vi "GeoData.vi"() -> ()   [LabVIEW 2017] (continued)
County\tH4\n1063\t25015\tNorthampton\tMA\tHampshire County\tH4\n1066\t25015\tNorth hatfield\tMA\tHampshire County\tH4\n1243\t25015\tMiddlefield\tMA\tHampshire County\tH4\n1007\t25015\tBelchertown\tMA\tHampshire County\tH4\n1011\t25015\tChester\tMA\tHampshire County\tH4\n1012\t25015\tChesterfield\tMA\tHampshire County\tH4\n1032\t25015\tGoshen\tMA\tHampshire County\tH4\n1027\t25015\tEasthampton\tMA\tHampshire County\tH4\n1060\t25015\tNorthampton\tMA\tHampshire County\tH4\n1033\t25015\tGranby\tMA\tHampshire County\tH4\n1038\t25015\tHatfield\tMA\tHampshire County\tH4\n1462\t25017\tLunenburg\tMA\tMiddlesex County\tH4\n1464\t25017\tShirley\tMA\tMiddlesex County\tH4\n1776\t25017\tSudbury\tMA\tMiddlesex County\tH4\n1803\t25017\tBurlington\tMA\tMiddlesex County\tH4\n1810\t25017\tAndover\tMA\tMiddlesex County\tH4\n1854\t25017\tLowell\tMA\tMiddlesex County\tH4\n1862\t25017\tNorth billerica\tMA\tMiddlesex County\tH4\n1879\t25017\tTyngsboro\tMA\tMiddlesex County\tH4\n2030\t25017\tDover\tMA\tMiddlesex County\tH4\n2054\t25017\tMillis\tMA\tMiddlesex County\tH4\n2143\t25017\tSomerville\tMA\tMiddlesex County\tH4\n2476\t25017\tArlington\tMA\tMiddlesex County\tH4\n1853\t25017\tLowell\tMA\tMiddlesex County\tH4\n1469\t25017\tTownsend\tMA\tMiddlesex County\tH4\n1703\t25017\tFramingham\tMA\tMiddlesex County\tH4\n1784\t25017\tWoodville\tMA\tMiddlesex County\tH4\n1805\t25017\tBurlington\tMA\tMiddlesex County\tH4\n1460\t25017\tLittleton\tMA\tMiddlesex County\tH4\n1746\t25017\tHolliston\tMA\tMiddlesex County\tH4\n1850\t25017\tLowell\tMA\tMiddlesex County\tH4\n1865\t25017\tNutting lake\tMA\tMiddlesex County\tH4\n1867\t25017\tReading\tMA\tMiddlesex County\tH4\n1876\t25017\tTewksbury\tMA\tMiddlesex County\tH4\n1880\t25017\tWakefield\tMA\tMiddlesex County\tH4\n1887\t25017\tWilmington\tMA\tMiddlesex County\tH4\n2149\t25017\tEverett\tMA\tMiddlesex County\tH4\n2238\t25017\tCambridge\tMA\tMiddlesex County\tH4\n2453\t25017\tWaltham\tMA\tMiddlesex County\tH4\n2454\t25017\tWaltham\tMA\tMiddlesex County\tH4\n2466\t25017\tAuburndale\tMA\tMiddlesex County\tH4\n1752\t25017\tMarlborough\tMA\tMiddlesex County\tH4\n1749\t25017\tHudson\tMA\tMiddlesex County\tH4\n1778\t25017\tWayland\tMA\tMiddlesex County\tH4\n2138\t25017\tCambridge\tMA\tMiddlesex County\tH4\n2142\t25017\tCambridge\tMA\tMiddlesex County\tH4\n2145\t25017\tSomerville\tMA\tMiddlesex County\tH4\n2151\t25017\tRevere\tMA\tMiddlesex County\tH4\n2452\t25017\tWaltham\tMA\tMiddlesex County\tH4\n2465\t25017\tWest newton\tMA\tMiddlesex County\tH4\n2461\t25017\tNewton highlands\tMA\tMiddlesex County\tH4\n2474\t25017\tArlington\tMA\tMiddlesex County\tH4\n2471\t25017\tWatertown\tMA\tMiddlesex County\tH4\n1718\t25017\tActon\tMA\tMiddlesex County\tH4\n1866\t25017\tPinehurst\tMA\tMiddlesex County\tH4\n1432\t25017\tAyer\tMA\tMiddlesex County\tH4\n1431\t25017\tAshby\tMA\tMiddlesex County\tH4\n1451\t25017\tHarvard\tMA\tMiddlesex County\tH4\n1701\t25017\tFramingham\tMA\tMiddlesex County\tH4\n1730\t25017\tBedford\tMA\tMiddlesex County\tH4\n1801\t25017\tWoburn\tMA\tMiddlesex County\tH4\n1822\t25017\tBillerica\tMA\tMiddlesex County\tH4\n2140\t25017\tCambridge\tMA\tMiddlesex County\tH4\n2459\t25017\tNewton center\tMA\tMiddlesex County\tH4\n1463\t25017\tPepperell\tMA\tMiddlesex County\tH4\n1474\t25017\tWest townsend\tMA\tMiddlesex County\tH4\n1720\t25017\tActon\tMA\tMiddlesex County\tH4\n1742\t25017\tConcord\tMA\tMiddlesex County\tH4\n1821\t25017\tBillerica\tMA\tMiddlesex County\tH4\n1851\t25017\tLowell\tMA\tMiddlesex County\tH4\n1863\t25017\tNorth chelmsford\tMA\tMiddlesex County\tH4\n2148\t25017\tMalden\tMA\tMiddlesex County\tH4\n2150\t25017\tChelsea\tMA\tMiddlesex County\tH4\n1741\t25017\tCarlisle\tMA\tMiddlesex County\tH4\n2462\t25017\tNewton lower falls\tMA\tMiddlesex County\tH4\n1472\t25017\tWest groton\tMA\tMiddlesex County\tH4\n2477\t25017\tWatertown\tMA\tMiddlesex County\tH4\n1532\t25017\tNorthborough\tMA\tMiddlesex County\tH4\n1721\t25017\tAshland\tMA\tMiddlesex County\tH4\n1748\t25017\tHopkinton\tMA\tMiddlesex County\tH4\n1760\t25017\tNatick\tMA\tMiddlesex County\tH4\n1770\t25017\tSherborn\tMA\tMiddlesex County\tH4\n1826\t25017\tDracut\tMA\tMiddlesex County\tH4\n1886\t25017\tWestford\tMA\tMiddlesex County\tH4\n2176\t25017\tMelrose\tMA\tMiddlesex County\tH4\n2451\t25017\tWaltham\tMA\tMiddlesex County\tH4\n2467\t25017\tChestnut hill\tMA\tMiddlesex County\tH4\n2478\t25017\tBelmont\tMA\tMiddlesex County\tH4\n1775\t25017\tStow\tMA\tMiddlesex County\tH4\n2464\t25017\tNewton upper falls\tMA\tMiddlesex County\tH4\n1824\t25017\tChelmsford\tMA\tMiddlesex County\tH4\n1827\t25017\tDunstable\tMA\tMiddlesex County\tH4\n1852\t25017\tLowell\tMA\tMiddlesex County\tH4\n1864\t25017\tNorth reading\tMA\tMiddlesex County\tH4\n2155\t25017\tMedford\tMA\tMiddlesex County\tH4\n2180\t25017\tStoneham\tMA\tMiddlesex County\tH4\n2420\t25017\tLexington\tMA\tMiddlesex County\tH4\n2460\t25017\tNewtonville\tMA\tMiddlesex County\tH4\n2472\t25017\tWatertown\tMA\tMiddlesex County\tH4\n2493\t25017\tWeston\tMA\tMiddlesex County\tH4\n1434\t25017\tDevens\tMA\tMiddlesex County\tH4\n1773\t25017\tLincoln\tMA\tMiddlesex County\tH4\n1888\t25017\tWoburn\tMA\tMiddlesex County\tH4\n2455\t25017\tNorth waltham\tMA\tMiddlesex County\tH4\n1450\t25017\tGroton\tMA\tMiddlesex County\tH4\n1702\t25017\tFramingham\tMA\tMiddlesex County\tH4\n1754\t25017\tMaynard\tMA\tMiddlesex County\tH4\n1890\t25017\tWinchester\tMA\tMiddlesex County\tH4\n1906\t25017\tSaugus\tMA\tMiddlesex County\tH4\n2139\t25017\tCambridge\tMA\tMiddlesex County\tH4\n2141\t25017\tCambridge\tMA\tMiddlesex County\tH4\n2144\t25017\tSomerville\tMA\tMiddlesex County\tH4\n2421\t25017\tLexington\tMA\tMiddlesex County\tH4\n2458\t25017\tNewton\tMA\tMiddlesex County\tH4\n1719\t25017\tBoxborough\tMA\tMiddlesex County\tH4\n2468\t25017\tWaban\tMA\tMiddlesex County\tH4\n1731\t25017\tHanscom afb\tMA\tMiddlesex County\tH4\n1704\t25017\tFramingham\tMA\tMiddlesex County\tH4\n1889\t25017\tNorth reading\tMA\tMiddlesex County\tH4\n2584\t25019\tNantucket\tMA\tNantucket County\tH4\n2564\t25019\tSiasconset\tMA\tNantucket County\tH4\n2554\t25019\tNantucket\tMA\tNantucket County\tH4\n2026\t25021\tDedham\tMA\tNorfolk County\tH1\n2030\t25021\tDover\tMA\tNorfolk County\tH1\n2035\t25021\tFoxboro\tMA\tNorfolk County\tH1\n2056\t25021\tNorfolk\tMA\tNorfolk County\tH1\n2062\t25021\tNorwood\tMA\tNorfolk County\tH1\n2054\t25021\tMillis\tMA\tNorfolk County\tH1\n2093\t25021\tWrentham\tMA\tNorfolk County\tH1\n2135\t25021\tBrighton\tMA\tNorfolk County\tH1\n2169\t25021\tQuincy\tMA\tNorfolk County\tH1\n2171\t25021\tQuincy\tMA\tNorfolk County\tH1\n2188\t25021\tWeymouth\tMA\tNorfolk County\tH1\n2482\t25021\tWellesley\tMA\tNorfolk County\tH1\n2762\t25021\tPlainville\tMA\tNorfolk County\tH1\n2027\t25021\tDedham\tMA\tNorfolk County\tH1\n2053\t25021\tMedway\tMA\tNorfolk County\tH1\n2269\t25021\tQuincy\tMA\tNorfolk County\tH1\n2185\t25021\tBraintree\tMA\tNorfolk County\tH1\n2070\t25021\tSheldonville\tMA\tNorfolk County\tH1\n2032\t25021\tEast walpole\tMA\tNorfolk County\tH1\n2130\t25021\tJamaica plain\tMA\tNorfolk County\tH1\n2215\t25021\tBoston\tMA\tNorfolk County\tH1\n2492\t25021\tNeedham\tMA\tNorfolk County\tH1\n2447\t25021\tBrookline village\tMA\tNorfolk County\tH1\n2038\t25021\tFranklin\tMA\tNorfolk County\tH1\n2067\t25021\tSharon\tMA\tNorfolk County\tH1\n2081\t25021\tWalpole\tMA\tNorfolk County\tH1\n2322\t25021\tAvon\tMA\tNorfolk County\tH1\n2071\t25021\tSouth walpole\tMA\tNorfolk County\tH1\n1504\t25021\tBlackstone\tMA\tNorfolk County\tH1\n2048\t25021\tMansfield\tMA\tNorfolk County\tH1\n2052\t25021\tMedfield\tMA\tNorfolk County\tH1\n2072\t25021\tStoughton\tMA\tNorfolk County\tH1\n2134\t25021\tAllston\tMA\tNorfolk County\tH1\n2189\t25021\tEast weymouth\tMA\tNorfolk County\tH1\n2302\t25021\tBrockton\tMA\tNorfolk County\tH1\n2481\t25021\tWellesley hills\tMA\tNorfolk County\tH1\n1760\t25021\tNatick\tMA\tNorfolk County\tH1\n2043\t25021\tHingham\tMA\tNorfolk County\tH1\n2066\t25021\tScituate\tMA\tNorfolk County\tH1\n2090\t25021\tWestwood\tMA\tNorfolk County\tH1\n2136\t25021\tHyde park\tMA\tNorfolk County\tH1\n2170\t25021\tQuincy\tMA\tNorfolk County\tH1\n2190\t25021\tSouth weymouth\tMA\tNorfolk County\tH1\n2368\t25021\tRandolph\tMA\tNorfolk County\tH1\n2467\t25021\tChestnut hill\tMA\tNorfolk County\tH1\n2464\t25021\tNewton upper falls\tMA\tNorfolk County\tH1\n2019\t25021\tBellingham\tMA\tNorfolk County\tH1\n2184\t25021\tBraintree\tMA\tNorfolk County\tH1\n2186\t25021\tMilton\tMA\tNorfolk County\tH1\n2191\t25021\tNorth weymouth\tMA\tNorfolk County\tH1\n2356\t25021\tNorth easton\tMA\tNorfolk County\tH1\n2445\t25021\tBrookline\tMA\tNorfolk County\tH1\n2446\t25021\tBrookline\tMA\tNorfolk County\tH1\n2021\t25021\tCanton\tMA\tNorfolk County\tH1\n2025\t25021\tCohasset\tMA\tNorfolk County\tH1\n2343\t25021\tHolbrook\tMA\tNorfolk County\tH1\n2494\t25021\tNeedham heights\tMA\tNorfolk County\tH1\n1756\t25021\tMendon\tMA\tNorfolk County\tH1\n2738\t25023\tMarion\tMA\tPlymouth County\tH1\n2770\t25023\tRochester\tMA\tPlymouth County\tH1\n2020\t25023\tBrant rock\tMA\tPlymouth County\tH1\n2051\t25023\tMarshfield hills\tMA\tPlymouth County\tH1\n2366\t25023\tSouth carver\tMA\tPlymouth County\tH1\n2381\t25023\tWhite horse beach\tMA\tPlymouth County\tH1\n2558\t25023\tOnset\tMA\tPlymouth County\tH1\n2344\t25023\tMiddleboro\tMA\tPlymouth County\tH1\n2050\t25023\tMarshfield\tMA\tPlymouth County\tH1\n2045\t25023\tHull\tMA\tPlymouth County\tH1\n2330\t25023\tCarver\tMA\tPlymouth County\tH1\n2324\t25023\tBridgewater\tMA\tPlymouth County\tH1\n2331\t25023\tDuxbury\tMA\tPlymouth County\tH1\n2346\t25023\tMiddleboro\tMA\tPlymouth County\tH1\n2351\t25023\tAbington\tMA\tPlymouth County\tH1\n2379\t25023\tWest bridgewater\tMA\tPlymouth County\tH1\n2702\t25023\tAssonet\tMA\tPlymouth County\tH1\n2041\t25023\tGreen harbor\tMA\tPlymouth County\tH1\n2361\t25023\tPlymouth\tMA\tPlymouth County\tH1\n2060\t25023\tNorth scituate\tMA\tPlymouth County\tH1\n2362\t25023\tPlymouth\tMA\tPlymouth County\tH1\n2348\t25023\tLakeville\tMA\tPlymouth County\tH1\n2327\t25023\tBryantville\tMA\tPlymouth County\tH1\n2061\t25023\tNorwell\tMA\tPlymouth County\tH1\n2333\t25023\tEast bridgewater\tMA\tPlymouth County\tH1\n2338\t25023\tHalifax\tMA\tPlymouth County\tH1\n2347\t25023\tLakeville\tMA\tPlymouth County\tH1\n2359\t25023\tPembroke\tMA\tPlymouth County\tH1\n2576\t25023\tWest wareham\tMA\tPlymouth County\tH1\n2303\t25023\tBrockton\tMA\tPlymouth County\tH1\n2349\t25023\tMiddleboro\tMA\tPlymouth County\tH1\n2382\t25023\tWhitman\tMA\tPlymouth County\tH1\n2532\t25023\tBuzzards bay\tMA\tPlymouth County\tH1\n2304\t25023\tBrockton\tMA\tPlymouth County\tH1\n2018\t25023\tAccord\tMA\tPlymouth County\tH1\n2358\t25023\tNorth pembroke\tMA\tPlymouth County\tH1\n2044\t25023\tHingham\tMA\tPlymouth County\tH1\n2189\t25023\tEast weymouth\tMA\tPlymouth County\tH1\n2302\t25023\tBrockton\tMA\tPlymouth County\tH1\n2305\t25023\tBrockton\tMA\tPlymouth County\tH1\n2779\t25023\tBerkley\tMA\tPlymouth County\tH1\n2043\t25023\tHingham\tMA\tPlymouth County\tH1\n2066\t25023\tScituate\tMA\tPlymouth County\tH1\n2301\t25023\tBrockton\tMA\tPlymouth County\tH1\n2341\t25023\tHanson\tMA\tPlymouth County\tH1\n2360\t25023\tPlymouth\tMA\tPlymouth County\tH1\n2370\t25023\tRockland\tMA\tPlymouth County\tH1\n2739\t25023\tMattapoisett\tMA\tPlymouth County\tH1\n2767\t25023\tRaynham\tMA\tPlymouth County\tH1\n2355\t25023\tNorth carver\tMA\tPlymouth County\tH1\n2332\t25023\tDuxbury\tMA\tPlymouth County\tH1\n2364\t25023\tKingston\tMA\tPlymouth County\tH1\n2367\t25023\tPlympton\tMA\tPlymouth County\tH1\n2375\t25023\tSouth easton\tMA\tPlymouth County\tH1\n2571\t25023\tWareham\tMA\tPlymouth County\tH1\n2059\t25023\tNorth marshfield\tMA\tPlymouth County\tH1\n2325\t25023\tBridgewater\tMA\tPlymouth County\tH1\n2337\t25023\tElmwood\tMA\tPlymouth County\tH1\n2025\t25023\tCohasset\tMA\tPlymouth County\tH1\n2047\t25023\tHumarock\tMA\tPlymouth County\tH1\n2339\t25023\tHanover\tMA\tPlymouth County\tH1\n2538\t25023\tEast wareham\tMA\tPlymouth County\tH1\n2345\t25023\tManomet\tMA\tPlymouth County\tH1\n2350\t25023\tMonponsett\tMA\tPlymouth County\tH1\n2065\t25023\tOcean bluff\tMA\tPlymouth County\tH1\n2026\t25025\tDedham\tMA\tSuffolk County\tH4\n2108\t25025\tBoston\tMA\tSuffolk County\tH4\n2113\t25025\tBoston\tMA\tSuffolk County\tH4\n2135\t25025\tBrighton\tMA\tSuffolk County\tH4\n2143\t25025\tSomerville\tMA\tSuffolk County\tH4\n2163\t25025\tBoston\tMA\tSuffolk County\tH4\n2201\t25025\tBoston\tMA\tSuffolk County\tH4\n2137\t25025\tReadville\tMA\tSuffolk County\tH4\n2109\t25025\tBoston\tMA\tSuffolk County\tH4\n2110\t25025\tBoston\tMA\tSuffolk County\tH4\n2111\t25025\tBoston\tMA\tSuffolk County\tH4\n2115\t25025\tBoston\tMA\tSuffolk County\tH4\n2124\t25025\tDorchester center\tMA\tSuffolk County\tH4\n2120\t25025\tRoxbury crossing\tMA\tSuffolk County\tH4\n2130\t25025\tJamaica plain\tMA\tSuffolk County\tH4\n2129\t25025\tCharlestown\tMA\tSuffolk County\tH4\n2151\t25025\tRevere\tMA\tSuffolk County\tH4\n2215\t25025\tBoston\tMA\tSuffolk County\tH4\n2196\t25025\tBoston\tMA\tSuffolk County\tH4\n2117\t25025\tBoston\tMA\tSuffolk County\tH4\n2122\t25025\tDorchester\tMA\tSuffolk County\tH4\n2126\t25025\tMattapan\tMA\tSuffolk County\tH4\n2125\t25025\tDorchester\tMA\tSuffolk County\tH4\n2127\t25025\tSouth boston\tMA\tSuffolk County\tH4\n2132\t25025\tWest roxbury\tMA\tSuffolk County\tH4\n2133\t25025\tBoston\tMA\tSuffolk County\tH4\n2203\t25025\tBoston\tMA\tSuffolk County\tH4\n2217\t25025\tBoston\tMA\tSuffolk County\tH4\n2118\t25025\tBoston\tMA\tSuffolk County\tH4\n2134\t25025\tAllston\tMA\tSuffolk County\tH4\n2148\t25025\tMalden\tMA\tSuffolk County\tH4\n2150\t25025\tChelsea\tMA\tSuffolk County\tH4\n2152\t25025\tWinthrop\tMA\tSuffolk County\tH4\n2136\t25025\tHyde park\tMA\tSuffolk County\tH4\n2210\t25025\tBoston\tMA\tSuffolk County\tH4\n2467\t25025\tChestnut hill\tMA\tSuffolk County\tH4\n2222\t25025\tBoston\tMA\tSuffolk County\tH4\n2119\t25025\tRoxbury\tMA\tSuffolk County\tH4\n2128\t25025\tEast boston\tMA\tSuffolk County\tH4\n2186\t25025\tMilton\tMA\tSuffolk County\tH4\n2445\t25025\tBrookline\tMA\tSuffolk County\tH4\n2446\t25025\tBrookline\tMA\tSuffolk County\tH4\n2205\t25025\tBoston\tMA\tSuffolk County\tH4\n1906\t25025\tSaugus\tMA\tSuffolk County\tH4\n2114\t25025\tBoston\tMA\tSuffolk County\tH4\n2112\t25025\tBoston\tMA\tSuffolk County\tH4\n2116\t25025\tBoston\tMA\tSuffolk County\tH4\n2121\t25025\tDorchester\tMA\tSuffolk County\tH4\n2123\t25025\tBoston\tMA\tSuffolk County\tH4\n2131\t25025\tRoslindale\tMA\tSuffolk County\tH4\n2199\t25025\tBoston\tMA\tSuffolk County\tH4\n1436\t25027\tBaldwinville\tMA\tWorcester County\tH4\n1462\t25027\tLunenburg\tMA\tWorcester County\tH4\n1516\t25027\tDouglas\tMA\tWorcester County\tH4\n1522\t25027\tJefferson\tMA\tWorcester County\tH4\n1569\t25027\tUxbridge\tMA\tWorcester County\tH4\n1581\t25027\tWestborough\tMA\tWorcester County\tH4\n1602\t25027\tWorcester\tMA\tWorcester County\tH4\n1606\t25027\tWorcester\tMA\tWorcester County\tH4\n1609\t25027\tWorcester\tMA\tWorcester County\tH4\n1757\t25027\tMilford\tMA\tWorcester County\tH4\n1655\t25027\tWorcester\tMA\tWorcester County\tH4\n1037\t25027\tHardwick\tMA\tWorcester County\tH4\n1509\t25027\tCharlton depot\tMA\tWorcester County\tH4\n1460\t25027\tLittleton\tMA\tWorcester County\tH4\n1568\t25027\tUpton\tMA\tWorcester County\tH4\n1570\t25027\tWebster\tMA\tWorcester County\tH4\n1608\t25027\tWorcester\tMA\tWorcester County\tH4\n1747\t25027\tHopedale\tMA\tWorcester County\tH4\n1537\t25027\tNorth oxford\tMA\tWorcester County\tH4\n1074\t25027\tSouth barre\tMA\tWorcester County\tH4\n1546\t25027\tShrewsbury\tMA\tWorcester County\tH4\n1561\t25027\tSouth lancaster\tMA\tWorcester County\tH4\n1441\t25027\tWestminster\tMA\tWorcester County\tH4\n1452\t25027\tHubbardston\tMA\tWorcester County\tH4\n1475\t25027\tWinchendon\tMA\tWorcester County\tH4\n1510\t25027\tClinton\tMA\tWorcester County\tH4\n1520\t25027\tHolden\tMA\tWorcester County\tH4\n1540\t25027\tOxford\tMA\tWorcester County\tH4\n1588\t25027\tWhitinsville\tMA\tWorcester County\tH4\n1585\t25027\tWest brookfield\tMA\tWorcester County\tH4\n1590\t25027\tSutton\tMA\tWorcester County\tH4\n1612\t25027\tPaxton\tMA\tWorcester County\tH4\n1613\t25027\tWorcester\tMA\tWorcester County\tH4\n1749\t25027\tHudson\tMA\tWorcester County\tH4\n1005\t25027\tBarre\tMA\tWorcester County\tH4\n1083\t25027\tWarren\tMA\tWorcester County\tH4\n1473\t25027\tWestminster\tMA\tWorcester County\tH4\n1368\t25027\tRoyalston\tMA\tWorcester County\tH4\n1506\t25027\tBrookfield\tMA\tWorcester County\tH4\n1468\t25027\tTempleton\tMA\tWorcester County\tH4\n1438\t25027\tEast templeton\tMA\tWorcester County\tH4\n1431\t25027\tAshby\tMA\tWorcester County\tH4\n1451\t25027\tHarvard\tMA\tWorcester County\tH4\n1507\t25027\tCharlton\tMA\tWorcester County\tH4\n1524\t25027\tLeicester\tMA\tWorcester County\tH4\n1543\t25027\tRutland\tMA\tWorcester County\tH4\n1545\t25027\tShrewsbury\tMA\tWorcester County\tH4\n1583\t25027\tWest boylston\tMA\tWorcester County\tH4\n1068\t25027\tOakham\tMA\tWorcester County\tH4\n1505\t25027\tBoylston\tMA\tWorcester County\tH4\n1745\t25027\tFayville\tMA\tWorcester County\tH4\n1094\t25027\tWheelwright\tMA\tWorcester County\tH4\n1420\t25027\tFitchburg\tMA\tWorcester County\tH4\n1440\t25027\tGardner\tMA\tWorcester County\tH4\n1504\t25027\tBlackstone\tMA\tWorcester County\tH4\n1503\t25027\tBerlin\tMA\tWorcester County\tH4\n1535\t25027\tNorth brookfield\tMA\tWorcester County\tH4\n1542\t25027\tRochdale\tMA\tWorcester County\tH4\n1571\t25027\tDudley\tMA\tWorcester County\tH4\n1610\t25027\tWorcester\tMA\tWorcester County\tH4\n1740\t25027\tBolton\tMA\tWorcester County\tH4\n1772\t25027\tSouthborough\tMA\tWorcester County\tH4\n1082\t25027\tWare\tMA\tWorcester County\tH4\n1518\t25027\tFiskdale\tMA\tWorcester County\tH4\n1508\t25027\tCharlton city\tMA\tWorcester County\tH4\n1467\t25027\tStill river\tMA\tWorcester County\tH4\n1430\t25027\tAshburnham\tMA\tWorcester County\tH4\n1527\t25027\tMillbury\tMA\tWorcester County\tH4\n1523\t25027\tLancaster\tMA\tWorcester County\tH4\n1519\t25027\tGrafton\tMA\tWorcester County\tH4\n1532\t25027\tNorthborough\tMA\tWorcester County\tH4\n1534\t25027\tNorthbridge\tMA\tWorcester County\tH4\n1605\t25027\tWorcester\tMA\tWorcester County\tH4\n1748\t25027\tHopkinton\tMA\tWorcester County\tH4\n1331\t25027\tAthol\tMA\tWorcester County\tH4\n1364\t25027\tOrange\tMA\tWorcester County\tH4\n1601\t25027\tWorcester\tMA\tWorcester County\tH4\n1010\t25027\tBrimfield\tMA\tWorcester County\tH4\n1653\t25027\tWorcester\tMA\tWorcester County\tH4\n1501\t25027\tAuburn\tMA\tWorcester County\tH4\n1550\t25027\tSouthbridge\tMA\tWorcester County\tH4\n1564\t25027\tSterling\tMA\tWorcester County\tH4\n1604\t25027\tWorcester\tMA\tWorcester County\tH4\n1607\t25027\tWorcester\tMA\tWorcester County\tH4\n1434\t25027\tDevens\tMA\tWorcester County\tH4\n1031\t25027\tGilbertville\tMA\tWorcester County\tH4\n1538\t25027\tNorth uxbridge\tMA\tWorcester County\tH4\n1092\t25027\tWest warren\tMA\tWorcester County\tH4\n1614\t25027\tWorcester\tMA\tWorcester County\tH4\n1526\t25027\tManchaug\tMA\tWorcester County\tH4\n1453\t25027\tLeominster\tMA\tWorcester County\tH4\n1529\t25027\tMillville\tMA\tWorcester County\tH4\n1560\t25027\tSouth grafton\tMA\tWorcester County\tH4\n1562\t25027\tSpencer\tMA\tWorcester County\tH4\n1566\t25027\tSturbridge\tMA\tWorcester County\tH4\n1603\t25027\tWorcester\tMA\tWorcester County\tH4\n1611\t25027\tCherry valley\tMA\tWorcester County\tH4\n1531\t25027\tNew braintree\tMA\tWorcester County\tH4\n1536\t25027\tNorth grafton\tMA\tWorcester County\tH4\n1541\t25027\tPrinceton\tMA\tWorcester County\tH4\n1756\t25027\tMendon\tMA\tWorcester County\tH4\n1515\t25027\tEast brookfield\tMA\tWorcester County\tH4\n1525\t25027\tLinwood\tMA\tWorcester County\tH4\n1366\t25027\tPetersham\tMA\tWorcester County\tH4\n1586\t25027\tWest millbury\tMA\tWorcester County\tH4\n48728\t26001\tCurran\tMI\tAlcona County\tH1\n48750\t26001\tOscoda\tMI\tAlcona County\tH1\n48721\t26001\tBlack river\tMI\tAlcona County\tH1\n49747\t26001\tHubbard lake\tMI\tAlcona County\tH1\n48742\t26001\tLincoln\tMI\tAlcona County\tH1\n48705\t26001\tBarton city\tMI\tAlcona County\tH1\n48762\t26001\tSpruce\tMI\tAlcona County\tH1\n48761\t26001\tSouth branch\tMI\tAlcona County\tH1\n48745\t26001\tMikado\tMI\tAlcona County\tH1\n48738\t26001\tGreenbush\tMI\tAlcona County\tH1\n48737\t26001\tGlennie\tMI\tAlcona County\tH1\n48740\t26001\tHarrisville\tMI\tAlcona County\tH1\n49891\t26003\tTrenary\tMI\tAlger County\tH1\n49816\t26003\tChatham\tMI\tAlger County\tH1\n49878\t26003\tRapid river\tMI\tAlger County\tH1\n49862\t26003\tMunising\tMI\tAlger County\tH1\n49885\t26003\tSkandia\tMI\tAlger County\tH1\n49839\t26003\tGrand marais\tMI\tAlger County\tH1\n49895\t26003\tWetmore\tMI\tAlger County\tH1\n49806\t26003\tAu train\tMI\tAlger County\tH1\n49883\t26003\tSeney\tMI\tAlger County\tH1\n49826\t26003\tRumely\tMI\tAlger County\tH1\n49884\t26003\tShingleton\tMI\tAlger County\tH1\n49825\t26003\tEben junction\tMI\tAlger County\tH1\n49822\t26003\tDeerton\tMI\tAlger County\tH1\n49080\t26005\tPlainwell\tMI\tAllegan County\tH1\n49323\t26005\tDorr\tMI\tAllegan County\tH1\n49423\t26005\tHolland\tMI\tAllegan County\tH1\n49426\t26005\tHudsonville\tMI\tAllegan County\tH1\n49026\t26005\tBloomingdale\tMI\tAllegan County\tH1\n49090\t26005\tSouth haven\tMI\tAllegan County\tH1\n49056\t26005\tGrand junction\tMI\tAllegan County\tH1\n49348\t26005\tWayland\tMI\tAllegan County\tH1\n49344\t26005\tShelbyville\tMI\tAllegan County\tH1\n49453\t26005\tSaugatuck\tMI\tAllegan County\tH1\n49315\t26005\tByron center\tMI\tAllegan County\tH1\n49316\t26005\tCaledonia\tMI\tAllegan County\tH1\n49419\t26005\tHamilton\tMI\tAllegan County\tH1\n49464\t26005\tZeeland\tMI\tAllegan County\tH1\n49070\t26005\tMartin\tMI\tAllegan County\tH1\n49406\t26005\tDouglas\tMI\tAllegan County\tH1\n49078\t26005\tOtsego\tMI\tAllegan County\tH1\n49328\t26005\tHopkins\tMI\tAllegan County\tH1\n49408\t26005\tFennville\tMI\tAllegan County\tH1\n49335\t26005\tMoline\tMI\tAllegan County\tH1\n49010\t26005\tAllegan\tMI\tAllegan County\tH1\n49333\t26005\tMiddleville\tMI\tAllegan County\tH1\n49055\t26005\tGobles\tMI\tAllegan County\tH1\n49450\t26005\tPullman\tMI\tAllegan County\tH1\n49416\t26005\tGlenn\tMI\tAllegan County\tH1\n49311\t26005\tBradley\tMI\tAllegan County\tH1\n49314\t26005\tBurnips\tMI\tAllegan County\tH1\n49744\t26007\tHerron\tMI\tAlpena County\tH1\n49747\t26007\tHubbard lake\tMI\tAlpena County\tH1\n48762\t26007\tSpruce\tMI\tAlpena County\tH1\n49753\t26007\tLachine\tMI\tAlpena County\tH1\n49707\t26007\tAlpena\tMI\tAlpena County\tH1\n49746\t26007\tHillman\tMI\tAlpena County\tH1\n49776\t26007\tPosen\tMI\tAlpena County\tH1\n49766\t26007\tOssineke\tMI\tAlpena County\tH1\n49729\t26009\tEllsworth\tMI\tAntrim County\tH1\n49690\t26009\tWilliamsburg\tMI\tAntrim County\tH1\n49612\t26009\tAlden\tMI\tAntrim County\tH1\n49629\t26009\tElk rapids\tMI\tAntrim County\tH1\n49615\t26009\tBellaire\tMI\tAntrim County\tH1\n49727\t26009\tEast jordan\tMI\tAntrim County\tH1\n49648\t26009\tKewadin\tMI\tAntrim County\tH1\n49622\t26009\tCentral lake\tMI\tAntrim County\tH1\n49659\t26009\tMancelona\tMI\tAntrim County\tH1\n49712\t26009\tBoyne city\tMI\tAntrim County\tH1\n49713\t26009\tBoyne falls\tMI\tAntrim County\tH1\n49730\t26009\tElmira\tMI\tAntrim County\tH1\n49627\t26009\tEastport\tMI\tAntrim County\tH1\n49720\t26009\tCharlevoix\tMI\tAntrim County\tH1\n49676\t26009\tRapid city\tMI\tAntrim County\tH1\n49611\t26009\tAlba\tMI\tAntrim County\tH1\n48650\t26011\tPinconning\tMI\tArenac County\tH1\n48770\t26011\tWhittemore\tMI\tArenac County\tH1\n48756\t26011\tPrescott\tMI\tArenac County\tH1\n48659\t26011\tSterling\tMI\tArenac County\tH1\n48766\t26011\tTwining\tMI\tArenac County\tH1\n48658\t26011\tStandish\tMI\tArenac County\tH1\n48613\t26011\tBentley\tMI\tArenac County\tH1\n48610\t26011\tAlger\tMI\tArenac County\tH1\n48765\t26011\tTurner\tMI\tArenac County\tH1\n48703\t26011\tAu gres\tMI\tArenac County\tH1\n48763\t26011\tTawas city\tMI\tArenac County\tH1\n48749\t26011\tOmer\tMI\tArenac County\tH1\n49946\t26013\tLanse\tMI\tBaraga County\tH1\n49908\t26013\tBaraga\tMI\tBaraga County\tH1\n49952\t26013\tNisula\tMI\tBaraga County\tH1\n49958\t26013\tPelkie\tMI\tBaraga County\tH1\n49919\t26013\tCovington\tMI\tBaraga County\tH1\n49962\t26013\tSkanee\tMI\tBaraga County\tH1\n49861\t26013\tMichigamme\tMI\tBaraga County\tH1\n49970\t26013\tWatton\tMI\tBaraga County\tH1\n48849\t26015\tLake odessa\tMI\tBarry County\tH1\n49080\t26015\tPlainwell\tMI\tBarry County\tH1\n49073\t26015\tNashville\tMI\tBarry County\tH1\n49325\t26015\tFreeport\tMI\tBarry County\tH1\n49083\t26015\tRichland\tMI\tBarry County\tH1\n49046\t26015\tDelton\tMI\tBarry County\tH1\n49348\t26015\tWayland\tMI\tBarry County\tH1\n49344\t26015\tShelbyville\tMI\tBarry County\tH1\n49060\t26015\tHickory corners\tMI\tBarry County\tH1\n49316\t26015\tCaledonia\tMI\tBarry County\tH1\n48897\t26015\tWoodland\tMI\tBarry County\tH1\n49021\t26015\tBellevue\tMI\tBarry County\tH1\n49017\t26015\tBattle creek\tMI\tBarry County\tH1\n49012\t26015\tAugusta\tMI\tBarry County\tH1\n49058\t26015\tHastings\tMI\tBarry County\tH1\n49050\t26015\tDowling\tMI\tBarry County\tH1\n49333\t26015\tMiddleville\tMI\tBarry County\tH1\n49035\t26015\tCloverdale\tMI\tBarry County\tH1\n48642\t26017\tMidland\tMI\tBay County\tH1\n48706\t26017\tBay city\tMI\tBay County\tH1\n48611\t26017\tAuburn\tMI\tBay County\tH1\n48757\t26017\tReese\tMI\tBay County\tH1\n48623\t26017\tFreeland\tMI\tBay County\tH1\n48650\t26017\tPinconning\tMI\tBay County\tH1\n48710\t26017\tUniversity center\tMI\tBay County\tH1\n48634\t26017\tLinwood\tMI\tBay County\tH1\n48659\t26017\tSterling\tMI\tBay County\tH1\n48708\t26017\tBay city\tMI\tBay County\tH1\n48732\t26017\tEssexville\tMI\tBay County\tH1\n48658\t26017\tStandish\tMI\tBay County\tH1\n48604\t26017\tSaginaw\tMI\tBay County\tH1\n48613\t26017\tBentley\tMI\tBay County\tH1\n48707\t26017\tBay city\tMI\tBay County\tH1\n48747\t26017\tMunger\tMI\tBay County\tH1\n48631\t26017\tKawkawlin\tMI\tBay County\tH1\n48652\t26017\tRhodes\tMI\tBay County\tH1\n49617\t26019\tBeulah\tMI\tBenzie County\tH1\n49650\t26019\tLake ann\tMI\tBenzie County\tH1\n49635\t26019\tFrankfort\tMI\tBenzie County\tH1\n49664\t26019\tMaple city\tMI\tBenzie County\tH1\n49628\t26019\tElberta\tMI\tBenzie County\tH1\n49640\t26019\tHonor\tMI\tBenzie County\tH1\n49643\t26019\tInterlochen\tMI\tBenzie County\tH1\n49616\t26019\tBenzonia\tMI\tBenzie County\tH1\n49684\t26019\tTraverse city\tMI\tBenzie County\tH1\n49613\t26019\tArcadia\tMI\tBenzie County\tH1\n49683\t26019\tThompsonville\tMI\tBenzie County\tH1\n49630\t26019\tEmpire\tMI\tBenzie County\tH1\n49120\t26021\tNiles\tMI\tBerrien County\tH1\n49127\t26021\tStevensville\tMI\tBerrien County\tH1\n49106\t26021\tBridgman\tMI\tBerrien County\tH1\n49043\t26021\tCovert\tMI\tBerrien County\tH1\n49047\t26021\tDowagiac\tMI\tBerrien County\tH1\n49113\t26021\tGalien\tMI\tBerrien County\tH1\n49111\t26021\tEau claire\tMI\tBerrien County\tH1\n49129\t26021\tUnion pier\tMI\tBerrien County\tH1\n49115\t26021\tHarbert\tMI\tBerrien County\tH1\n49104\t26021\tBerrien springs\tMI\tBerrien County\tH1\n49107\t26021\tBuchanan\tMI\tBerrien County\tH1\n49098\t26021\tWatervliet\tMI\tBerrien County\tH1\n49126\t26021\tSodus\tMI\tBerrien County\tH1\n49084\t26021\tRiverside\tMI\tBerrien County\tH1\n49022\t26021\tBenton harbor\tMI\tBerrien County\tH1\n49102\t26021\tBerrien center\tMI\tBerrien County\tH1\n49119\t26021\tNew troy\tMI\tBerrien County\tH1\n49128\t26021\tThree oaks\tMI\tBerrien County\tH1\n49101\t26021\tBaroda\tMI\tBerrien County\tH1\n49117\t26021\tNew buffalo\tMI\tBerrien County\tH1\n49116\t26021\tLakeside\tMI\tBerrien County\tH1\n49038\t26021\tColoma\tMI\tBerrien County\tH1\n49103\t26021\tBerrien springs\tMI\tBerrien County\tH1\n49125\t26021\tSawyer\tMI\tBerrien County\tH1\n49085\t26021\tSaint joseph\tMI\tBerrien County\tH1\n49023\t26021\tBenton harbor\tMI\tBerrien County\tH1\n49040\t26023\tColon\tMI\tBranch County\tH1\n49092\t26023\tTekonsha\tMI\tBranch County\tH1\n49255\t26023\tMontgomery\tMI\tBranch County\tH1\n49082\t26023\tQuincy\tMI\tBranch County\tH1\n49274\t26023\tReading\tMI\tBranch County\tH1\n49245\t26023\tHomer\tMI\tBranch County\tH1\n49036\t26023\tColdwater\tMI\tBranch County\tH1\n49011\t26023\tAthens\tMI\tBranch County\tH1\n49252\t26023\tLitchfield\tMI\tBranch County\tH1\n49227\t26023\tAllen\tMI\tBranch County\tH1\n49028\t26023\tBronson\tMI\tBranch County\tH1\n49089\t26023\tSherwood\tMI\tBranch County\tH1\n49030\t26023\tBurr oak\tMI\tBranch County\tH1\n49094\t26023\tUnion city\tMI\tBranch County\tH1\n49224\t26025\tAlbion\tMI\tCalhoun County\tH1\n49092\t26025\tTekonsha\tMI\tCalhoun County\tH1\n49245\t26025\tHomer\tMI\tCalhoun County\tH1\n49016\t26025\tBattle creek\tMI\tCalhoun County\tH1\n49076\t26025\tOlivet\tMI\tCalhoun County\tH1\n49011\t26025\tAthens\tMI\tCalhoun County\tH1\n49252\t26025\tLitchfield\tMI\tCalhoun County\tH1\n49284\t26025\tSpringport\tMI\tCalhoun County\tH1\n49237\t26025\tConcord\tMI\tCalhoun County\tH1\n49051\t26025\tEast leroy\tMI\tCalhoun County\tH1\n49034\t26025\tClimax\tMI\tCalhoun County\tH1\n49015\t26025\tBattle creek\tMI\tCalhoun County\tH1\n49068\t26025\tMarshall\tMI\tCalhoun County\tH1\n49052\t26025\tFulton\tMI\tCalhoun County\tH1\n49021\t26025\tBellevue\tMI\tCalhoun County\tH1\n48813\t26025\tCharlotte\tMI\tCalhoun County\tH1\n49014\t26025\tBattle creek\tMI\tCalhoun County\tH1\n49017\t26025\tBattle creek\tMI\tCalhoun County\tH1\n49029\t26025\tBurlington\tMI\tCalhoun County\tH1\n49037\t26025\tBattle creek\tMI\tCalhoun County\tH1\n49012\t26025\tAugusta\tMI\tCalhoun County\tH1\n49033\t26025\tCeresco\tMI\tCalhoun County\tH1\n49094\t26025\tUnion city\tMI\tCalhoun County\tH1\n49020\t26025\tBedford\tMI\tCalhoun County\tH1\n49031\t26027\tCassopolis\tMI\tCass County\tH1\n49099\t26027\tWhite pigeon\tMI\tCass County\tH1\n49120\t26027\tNiles\tMI\tCass County\tH1\n49112\t26027\tEdwardsburg\tMI\tCass County\tH1\n49047\t26027\tDowagiac\tMI\tCass County\tH1\n49111\t26027\tEau claire\tMI\tCass County\tH1\n49042\t26027\tConstantine\tMI\tCass County\tH1\n49045\t26027\tDecatur\tMI\tCass County\tH1\n49102\t26027\tBerrien center\tMI\tCass County\tH1\n49093\t26027\tThree rivers\tMI\tCass County\tH1\n49065\t26027\tLawton\tMI\tCass County\tH1\n49061\t26027\tJones\tMI\tCass County\tH1\n49067\t26027\tMarcellus\tMI\tCass County\tH1\n49130\t26027\tUnion\tMI\tCass County\tH1\n49095\t26027\tVandalia\tMI\tCass County\tH1\n49729\t26029\tEllsworth\tMI\tCharlevoix County\tH1\n49782\t26029\tBeaver island\tMI\tCharlevoix County\tH1\n49727\t26029\tEast jordan\tMI\tCharlevoix County\tH1\n49796\t26029\tWalloon lake\tMI\tCharlevoix County\tH1\n49795\t26029\tVanderbilt\tMI\tCharlevoix County\tH1\n49712\t26029\tBoyne city\tMI\tCharlevoix County\tH1\n49713\t26029\tBoyne falls\tMI\tCharlevoix County\tH1\n49770\t26029\tPetoskey\tMI\tCharlevoix County\tH1\n49730\t26029\tElmira\tMI\tCharlevoix County\tH1\n49720\t26029\tCharlevoix\tMI\tCharlevoix County\tH1\n49769\t26031\tPellston\tMI\tCheboygan County\tH1\n49718\t26031\tCarp lake\tMI\tCheboygan County\tH1\n49799\t26031\tWolverine\tMI\tCheboygan County\tH1\n49791\t26031\tTopinabee\tMI\tCheboygan County\tH1\n49749\t26031\tIndian river\tMI\tCheboygan County\tH1\n49701\t26031\tMackinaw city\tMI\tCheboygan County\tH1\n49706\t26031\tAlanson\tMI\tCheboygan County\tH1\n49716\t26031\tBrutus\tMI\tCheboygan County\tH1\n49795\t26031\tVanderbilt\tMI\tCheboygan County\tH1\n49717\t26031\tBurt lake\tMI\tCheboygan County\tH1\n49721\t26031\tCheboygan\tMI\tCheboygan County\tH1\n49761\t26031\tMullett lake\tMI\tCheboygan County\tH1\n49705\t26031\tAfton\tMI\tCheboygan County\tH1\n49770\t26031\tPetoskey\tMI\tCheboygan County\tH1\n49755\t26031\tLevering\tMI\tCheboygan County\tH1\n49792\t26031\tTower\tMI\tCheboygan County\tH1\n49765\t26031\tOnaway\tMI\tCheboygan County\tH1\n49783\t26033\tSault sainte marie\tMI\tChippewa County\tH1\n49710\t26033\tBarbeau\tMI\tChippewa County\tH1\n49780\t26033\tRudyard\tMI\tChippewa County\tH1\n49748\t26033\tHulbert\tMI\tChippewa County\tH1\n49868\t26033\tNewberry\tMI\tChippewa County\tH1\n49760\t26033\tMoran\tMI\tChippewa County\tH1\n49768\t26033\tParadise\tMI\tChippewa County\tH1\n49725\t26033\tDe tour village\tMI\tChippewa County\tH1\n49752\t26033\tKinross\tMI\tChippewa County\tH1\n49719\t26033\tCedarville\tMI\tChippewa County\tH1\n49793\t26033\tTrout lake\tMI\tChippewa County\tH1\n49724\t26033\tDafter\tMI\tChippewa County\tH1\n49728\t26033\tEckerman\tMI\tChippewa County\tH1\n49788\t26033\tKincheloe\tMI\tChippewa County\tH1\n49774\t26033\tPickford\tMI\tChippewa County\tH1\n49715\t26033\tBrimley\tMI\tChippewa County\tH1\n49726\t26033\tDrummond island\tMI\tChippewa County\tH1\n49736\t26033\tGoetzville\tMI\tChippewa County\tH1\n48632\t26035\tLake\tMI\tClare County\tH1\n48624\t26035\tGladwin\tMI\tClare County\tH1\n48612\t26035\tBeaverton\tMI\tClare County\tH1\n49665\t26035\tMarion\tMI\tClare County\tH1\n48633\t26035\tLake george\tMI\tClare County\tH1\n48625\t26035\tHarrison\tMI\tClare County\tH1\n48622\t26035\tFarwell\tMI\tClare County\tH1\n49679\t26035\tSears\tMI\tClare County\tH1\n48617\t26035\tClare\tMI\tClare County\tH1\n48840\t26037\tHaslett\tMI\tClinton County\tH1\n48875\t26037\tPortland\tMI\tClinton County\tH1\n48833\t26037\tEureka\tMI\tClinton County\tH1\n48951\t26037\tLansing\tMI\tClinton County\tH1\n48848\t26037\tLaingsburg\tMI\tClinton County\tH1\n48879\t26037\tSaint johns\tMI\tClinton County\tH1\n48873\t26037\tPewamo\tMI\tClinton County\tH1\n48820\t26037\tDewitt\tMI\tClinton County\tH1\n48845\t26037\tHubbardston\tMI\tClinton County\tH1\n48808\t26037\tBath\tMI\tClinton County\tH1\n48906\t26037\tLansing\tMI\tClinton County\tH1\n48835\t26037\tFowler\tMI\tClinton County\tH1\n48894\t26037\tWestphalia\tMI\tClinton County\tH1\n48853\t26037\tMaple rapids\tMI\tClinton County\tH1\n48823\t26037\tEast lansing\tMI\tClinton County\tH1\n48837\t26037\tGrand ledge\tMI\tClinton County\tH1\n48822\t26037\tEagle\tMI\tClinton County\tH1\n48866\t26037\tOvid\tMI\tClinton County\tH1\n48871\t26037\tPerrinton\tMI\tClinton County\tH1\n48807\t26037\tBannister\tMI\tClinton County\tH1\n48831\t26037\tElsie\tMI\tClinton County\tH1\n48653\t26039\tRoscommon\tMI\tCrawford County\tH1\n49738\t26039\tGrayling\tMI\tCrawford County\tH1\n49756\t26039\tLewiston\tMI\tCrawford County\tH1\n49733\t26039\tFrederic\tMI\tCrawford County\tH1\n49837\t26041\tGladstone\tMI\tDelta County\tH1\n49878\t26041\tRapid river\tMI\tDelta County\tH1\n49880\t26041\tRock\tMI\tDelta County\tH1\n49817\t26041\tCooks\tMI\tDelta County\tH1\n49807\t26041\tBark river\tMI\tDelta County\tH1\n49829\t26041\tEscanaba\tMI\tDelta County\tH1\n49835\t26041\tGarden\tMI\tDelta County\tH1\n49895\t26041\tWetmore\tMI\tDelta County\tH1\n49818\t26041\tCornell\tMI\tDelta County\tH1\n49894\t26041\tWells\tMI\tDelta County\tH1\n49872\t26041\tPerkins\tMI\tDelta County\tH1\n49854\t26041\tManistique\tMI\tDelta County\tH1\n49864\t26041\tNahma\tMI\tDelta County\tH1\n49801\t26043\tIron mountain\tMI\tDickinson County\tH1\n49834\t26043\tFoster city\tMI\tDickinson County\tH1\n49870\t26043\tNorway\tMI\tDickinson County\tH1\n49831\t26043\tFelch\tMI\tDickinson County\tH1\n49852\t26043\tLoretto\tMI\tDickinson County\tH1\n49920\t26043\tCrystal falls\tMI\tDickinson County\tH1\n49815\t26043\tChanning\tMI\tDickinson County\tH1\n49881\t26043\tSagola\tMI\tDickinson County\tH1\n49876\t26043\tQuinnesec\tMI\tDickinson County\tH1\n49873\t26043\tPerronville\tMI\tDickinson County\tH1\n49802\t26043\tKingsford\tMI\tDickinson County\tH1\n49892\t26043\tVulcan\tMI\tDickinson County\tH1\n49877\t26043\tRalph\tMI\tDickinson County\tH1\n48849\t26045\tLake odessa\tMI\tEaton County\tH1\n49073\t26045\tNashville\tMI\tEaton County\tH1\n48908\t26045\tLansing\tMI\tEaton County\tH1\n49076\t26045\tOlivet\tMI\tEaton County\tH1\n48821\t26045\tDimondale\tMI\tEaton County\tH1\n48890\t26045\tSunfield\tMI\tEaton County\tH1\n48876\t26045\tPotterville\tMI\tEaton County\tH1\n48911\t26045\tLansing\tMI\tEaton County\tH1\n48917\t26045\tLansing\tMI\tEaton County\tH1\n49284\t26045\tSpringport\tMI\tEaton County\tH1\n48842\t26045\tHolt\tMI\tEaton County\tH1\n48897\t26045\tWoodland\tMI\tEaton County\tH1\n48906\t26045\tLansing\tMI\tEaton County\tH1\n49096\t26045\tVermontville\tMI\tEaton County\tH1\n49021\t26045\tBellevue\tMI\tEaton County\tH1\n49264\t26045\tOnondaga\tMI\tEaton County\tH1\n48837\t26045\tGrand ledge\tMI\tEaton County\tH1\n48813\t26045\tCharlotte\tMI\tEaton County\tH1\n49014\t26045\tBattle creek\tMI\tEaton County\tH1\n48861\t26045\tMulliken\tMI\tEaton County\tH1\n48827\t26045\tEaton rapids\tMI\tEaton County\tH1\n49769\t26047\tPellston\tMI\tEmmet County\tH1\n49718\t26047\tCarp lake\tMI\tEmmet County\tH1\n49799\t26047\tWolverine\tMI\tEmmet County\tH1\n49764\t26047\tOden\tMI\tEmmet County\tH1\n49722\t26047\tConway\tMI\tEmmet County\tH1\n49701\t26047\tMackinaw city\tMI\tEmmet County\tH1\n49723\t26047\tCross village\tMI\tEmmet County\tH1\n49740\t26047\tHarbor springs\tMI\tEmmet County\tH1\n49706\t26047\tAlanson\tMI\tEmmet County\tH1\n49716\t26047\tBrutus\tMI\tEmmet County\tH1\n49713\t26047\tBoyne falls\tMI\tEmmet County\tH1\n49770\t26047\tPetoskey\tMI\tEmmet County\tH1\n49755\t26047\tLevering\tMI\tEmmet County\tH1\n49720\t26047\tCharlevoix\tMI\tEmmet County\tH1\n48462\t26049\tOrtonville\tMI\tGenesee County\tH1\n48420\t26049\tClio\tMI\tGenesee County\tH1\n48421\t26049\tColumbiaville\tMI\tGenesee County\tH1\n48503\t26049\tFlint\tMI\tGenesee County\tH1\n48442\t26049\tHolly\tMI\tGenesee County\tH1\n48458\t26049\tMount morris\tMI\tGenesee County\tH1\n48417\t26049\tBurt\tMI\tGenesee County\tH1\n48501\t26049\tFlint\tMI\tGenesee County\tH1\n48550\t26049\tFlint\tMI\tGenesee County\tH1\n48505\t26049\tFlint\tMI\tGenesee County\tH1\n48451\t26049\tLinden\tMI\tGenesee County\tH1\n48746\t26049\tMillington\tMI\tGenesee County\tH1\n48430\t26049\tFenton\tMI\tGenesee County\tH1\n48429\t26049\tDurand\tMI\tGenesee County\tH1\n48457\t26049\tMontrose\tMI\tGenesee County\tH1\n48504\t26049\tFlint\tMI\tGenesee County\tH1\n48532\t26049\tFlint\tMI\tGenesee County\tH1\n48438\t26049\tGoodrich\tMI\tGenesee County\tH1\n48418\t26049\tByron\tMI\tGenesee County\tH1\n48506\t26049\tFlint\tMI\tGenesee County\tH1\n48529\t26049\tBurton\tMI\tGenesee County\tH1\n48507\t26049\tFlint\tMI\tGenesee County\tH1\n48464\t26049\tOtter lake\tMI\tGenesee County\tH1\n48463\t26049\tOtisville\tMI\tGenesee County\tH1\n48415\t26049\tBirch run\tMI\tGenesee County\tH1\n48439\t26049\tGrand blanc\tMI\tGenesee County\tH1\n48502\t26049\tFlint\tMI\tGenesee County\tH1\n48509\t26049\tBurton\tMI\tGenesee County\tH1\n48480\t26049\tGrand blanc\tMI\tGenesee County\tH1\n48519\t26049\tBurton\tMI\tGenesee County\tH1\n48473\t26049\tSwartz creek\tMI\tGenesee County\tH1\n48423\t26049\tDavison\tMI\tGenesee County\tH1\n48460\t26049\tNew lothrop\tMI\tGenesee County\tH1\n48433\t26049\tFlushing\tMI\tGenesee County\tH1\n48436\t26049\tGaines\tMI\tGenesee County\tH1\n48449\t26049\tLennon\tMI\tGenesee County\tH1\n48437\t26049\tGenesee\tMI\tGenesee County\tH1\n48531\t26049\tFlint\tMI\tGenesee County\tH1\n48411\t26049\tAtlas\tMI\tGenesee County\tH1\n48624\t26051\tGladwin\tMI\tGladwin County\tH1\n48628\t26051\tHope\tMI\tGladwin County\tH1\n48612\t26051\tBeaverton\tMI\tGladwin County\tH1\n48618\t26051\tColeman\tMI\tGladwin County\tH1\n48613\t26051\tBentley\tMI\tGladwin County\tH1\n48610\t26051\tAlger\tMI\tGladwin County\tH1\n48652\t26051\tRhodes\tMI\tGladwin County\tH1\n49938\t26053\tIronwood\tMI\tGogebic County\tH1\n49947\t26053\tMarenisco\tMI\tGogebic County\tH1\n49969\t26053\tWatersmeet\tMI\tGogebic County\tH1\n49968\t26053\tWakefield\tMI\tGogebic County\tH1\n49911\t26053\tBessemer\tMI\tGogebic County\tH1\n49959\t26053\tRamsay\tMI\tGogebic County\tH1\n49686\t26055\tTraverse city\tMI\tGrand Traverse County\tH1\n49620\t26055\tBuckley\tMI\tGrand Traverse County\tH1\n49690\t26055\tWilliamsburg\tMI\tGrand Traverse County\tH1\n49610\t26055\tAcme\tMI\tGrand Traverse County\tH1\n49633\t26055\tFife lake\tMI\tGrand Traverse County\tH1\n49637\t26055\tGrawn\tMI\tGrand Traverse County\tH1\n49685\t26055\tTraverse city\tMI\tGrand Traverse County\tH1\n49643\t26055\tInterlochen\tMI\tGrand Traverse County\tH1\n49673\t26055\tOld mission\tMI\tGrand Traverse County\t
